vi "LibXML_InitParser.vi"(8 "error in":errorcluster) -> (0 "error out":errorcluster)   [LabVIEW 2019, in "Tools.lvlib" / "LibXML.lvlib"]
doc: "Call once before processing in case of use in multithreaded programs."
uses:
  LibXML.lvlib
  dll/libxml2.dll
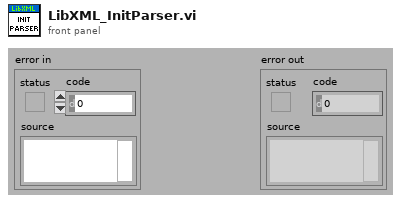
[diagram p1: front panel]
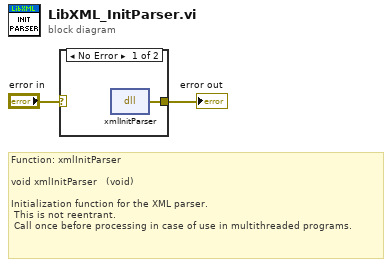
[diagram p0: block diagram]
diagram:
  # "Function: xmlInitParser\n\nvoid\txmlInitParser\t\t\t(void)\n\nInitialization function for the XML parser.\n This is not reentrant.\n Call once before processing in case of use in multithreaded programs."
  n1 = case shown="No Error" "error in" {
    selector: "error in" -> [_ w4]
    tunnel: [w3 w4] -> w1
    frame No Error {
      n2 = dll-call lib="C:/Projects/_Prywatne/MyCIT/Framework/Tools/XML/LibXML/dll/libxml2.dll" fn="xmlInitParser"() -> (error out=w3:errorcluster)  [unwired: 4 in, 1 out]
    }
    frame Error {
    }
  }
  "error out" <- w1
